vi "FL Get Rules as Text.vi"(8 "error in (no error)":errorcluster, 11 "fuzzy system in":T1 {"user MF interpolating polynomials"."coa_x(y) coeff" format="%.4g"; "user MF interpolating polynomials"."Area(y) coeff" format="%.4g"; "user MF interpolating polynomials"."X(y) coeff" format="%.4g"; "user MF interpolating polynomials"."Y(x) coeff" format="%.4g"; "user MF interpolating polynomials"."Y" format="%.4g"; "user MF interpolating polynomials"."X" format="%.4g"; "defuzzification method" items=["Center of Area", "Modified Center of Area", "Center of Sums", "Center of Maximum", "Mean of Maximum"]; "rules"."consequents"."Var Index" min=0; "rules"."consequents"."Cond" items=["=", "!="]; "rules"."consequents"."MF Index" min=0; "rules"."antecedents"."Var Index" min=0; "rules"."antecedents"."Cond" items=["=", "!="]; "rules"."antecedents"."MF Index" min=0; "rules"."consequent implication" items=["Minimum", "Product"]; "rules"."antecedent connective" items=["AND (Minimum)", "AND (Product)", "OR (Maximum)", "OR (Probabilistic)"]; "output variables"."MFs"."shape" items=["Triangle", "Trapezoid", "Singleton", "Sigmoid", "Gaussian", "User-Defined"]; "input variables"."MFs"."shape" items=["Triangle", "Trapezoid", "Singleton", "Sigmoid", "Gaussian", "User-Defined"]}) -> (0 "error out":errorcluster, 2 "rules as text":string[](array[string]), 3 "fuzzy system out":T1 {"user MF interpolating polynomials"."coa_x(y) coeff" format="%.4g"; "user MF interpolating polynomials"."Area(y) coeff" format="%.4g"; "user MF interpolating polynomials"."X(y) coeff" format="%.4g"; "user MF interpolating polynomials"."Y(x) coeff" format="%.4g"; "user MF interpolating polynomials"."Y" format="%.4g"; "user MF interpolating polynomials"."X" format="%.4g"; "defuzzification method" items=["Center of Area", "Modified Center of Area", "Center of Sums", "Center of Maximum", "Mean of Maximum"]; "rules"."consequents"."Var Index" min=0; "rules"."consequents"."Cond" items=["=", "!="]; "rules"."consequents"."MF Index" min=0; "rules"."antecedents"."Var Index" min=0; "rules"."antecedents"."Cond" items=["=", "!="]; "rules"."antecedents"."MF Index" min=0; "rules"."consequent implication" items=["Minimum", "Product"]; "rules"."antecedent connective" items=["AND (Minimum)", "AND (Product)", "OR (Maximum)", "OR (Probabilistic)"]; "output variables"."MFs"."shape" items=["Triangle", "Trapezoid", "Singleton", "Sigmoid", "Gaussian", "User-Defined"]; "input variables"."MFs"."shape" items=["Triangle", "Trapezoid", "Singleton", "Sigmoid", "Gaussian", "User-Defined"]})   [LabVIEW 2017, in "NI_Fuzzy_Logic_API.lvlib"]
doc: "Returns the rules of a fuzzy system in words."
uses:
  <vilib>/addons/Fuzzy Logic/NI_Fuzzy_Logic_API.lvlib
  <vilib>/addons/Fuzzy Logic/TypeDefs/FL System.ctl
  <vilib>/addons/Fuzzy Logic/TypeDefs/FL Variable.ctl
  <vilib>/addons/Fuzzy Logic/TypeDefs/FL Membership Function.ctl
  <vilib>/addons/Fuzzy Logic/TypeDefs/FL Membership Function Shape.ctl
  <vilib>/addons/Fuzzy Logic/TypeDefs/FL Rule.ctl
  <vilib>/addons/Fuzzy Logic/TypeDefs/FL Antecedent.ctl
  <vilib>/addons/Fuzzy Logic/TypeDefs/FL Modifier.ctl
  <vilib>/addons/Fuzzy Logic/TypeDefs/FL Antecedent Connective.ctl
  <vilib>/addons/Fuzzy Logic/TypeDefs/FL Consequent.ctl
  <vilib>/addons/Fuzzy Logic/TypeDefs/FL Consequent Implication.ctl
  <vilib>/addons/Fuzzy Logic/TypeDefs/FL Defuzzification.ctl
  <vilib>/addons/Fuzzy Logic/TypeDefs/FL Interpolating polynomials.ctl
panel:
  # "IF"
  # "THEN"
  # "IF"
  # "THEN"
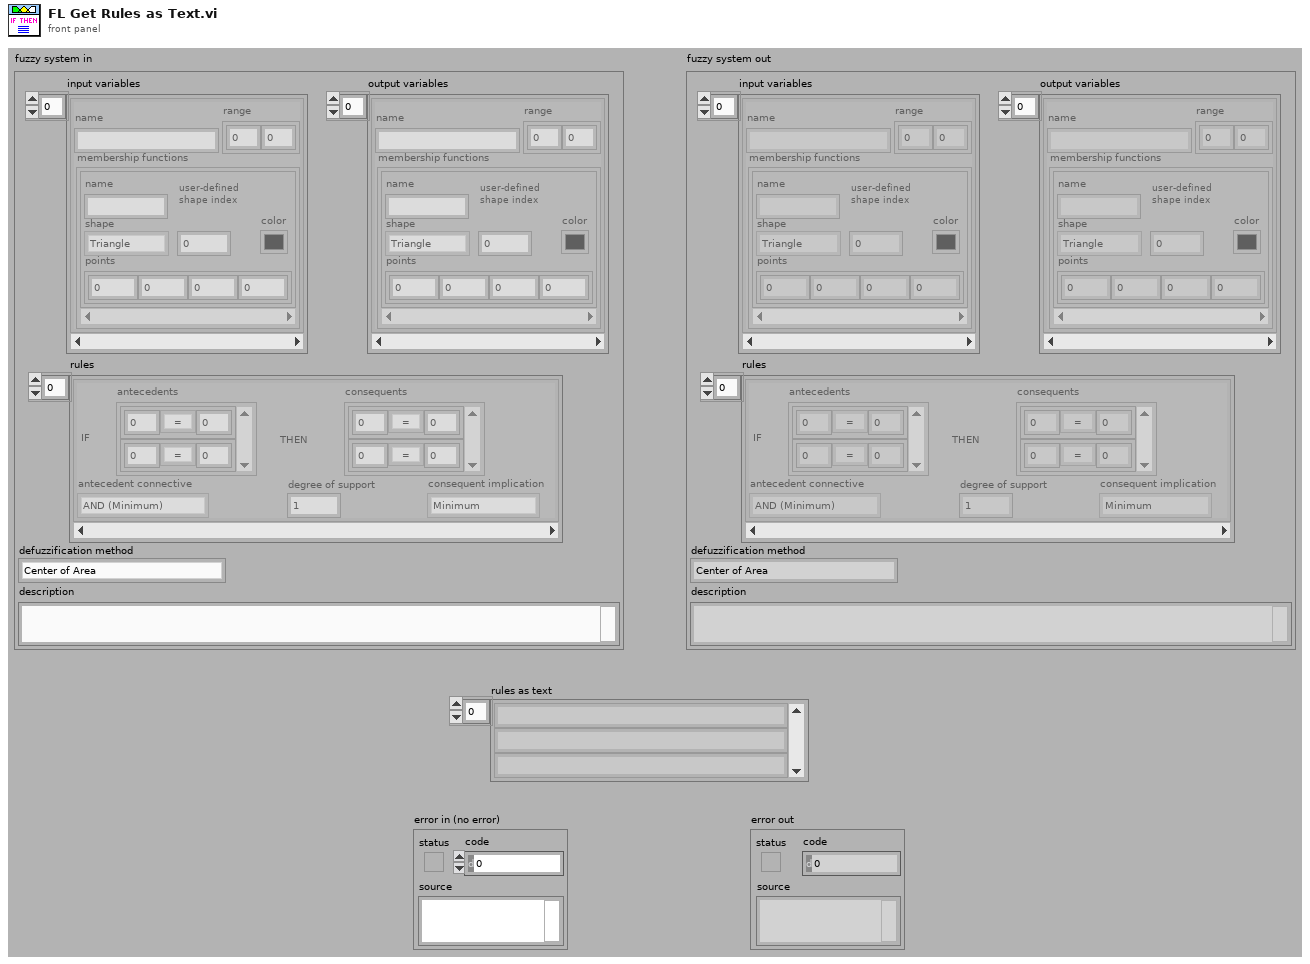
[diagram p1: front panel]
types:
  T1 = typedef "NI_Fuzzy_Logic_API.lvlib/FL System.ctl" = cluster{"input variables":T2[], "output variables":T2[], "rules":T5[], "defuzzification method":T11, "description":string, "user MF interpolating polynomials":T12[]}
  T2 = typedef "NI_Fuzzy_Logic_API.lvlib/FL Variable.ctl" = cluster{"name":string, "range":dbl[], "MFs":T3[]}
  T3 = typedef "NI_Fuzzy_Logic_API.lvlib/FL Membership Function.ctl" = cluster{"name":string, "shape":T4, "points":dbl[], "color":u32, "user-defined shape index":i32}
  T4 = typedef "NI_Fuzzy_Logic_API.lvlib/FL Membership Function Shape.ctl" = u16
  T5 = typedef "NI_Fuzzy_Logic_API.lvlib/FL Rule.ctl" = cluster{"antecedents":T6[], "antecedent connective":T8, "consequents":T9[], "consequent implication":T10, "degree of support":dbl}
  T6 = typedef "NI_Fuzzy_Logic_API.lvlib/FL Antecedent.ctl" = cluster{"Var Index":i32, "MF Index":i32, "Cond":T7}
  T7 = typedef "NI_Fuzzy_Logic_API.lvlib/FL Modifier.ctl" = u16
  T8 = typedef "NI_Fuzzy_Logic_API.lvlib/FL Antecedent Connective.ctl" = u16
  T9 = typedef "NI_Fuzzy_Logic_API.lvlib/FL Consequent.ctl" = cluster{"Var Index":i32, "MF Index":i32, "Cond":T7}
  T10 = typedef "NI_Fuzzy_Logic_API.lvlib/FL Consequent Implication.ctl" = u16
  T11 = typedef "NI_Fuzzy_Logic_API.lvlib/FL Defuzzification.ctl" = u16
  T12 = typedef "NI_Fuzzy_Logic_API.lvlib/FL Interpolating polynomials.ctl" = cluster{"X":dbl[], "Y":dbl[], "Y(x) coeff":dbl[][], "X(y) coeff":dbl[][], "Area(y) coeff":dbl[][], "coa_x(y) coeff":dbl[][]}
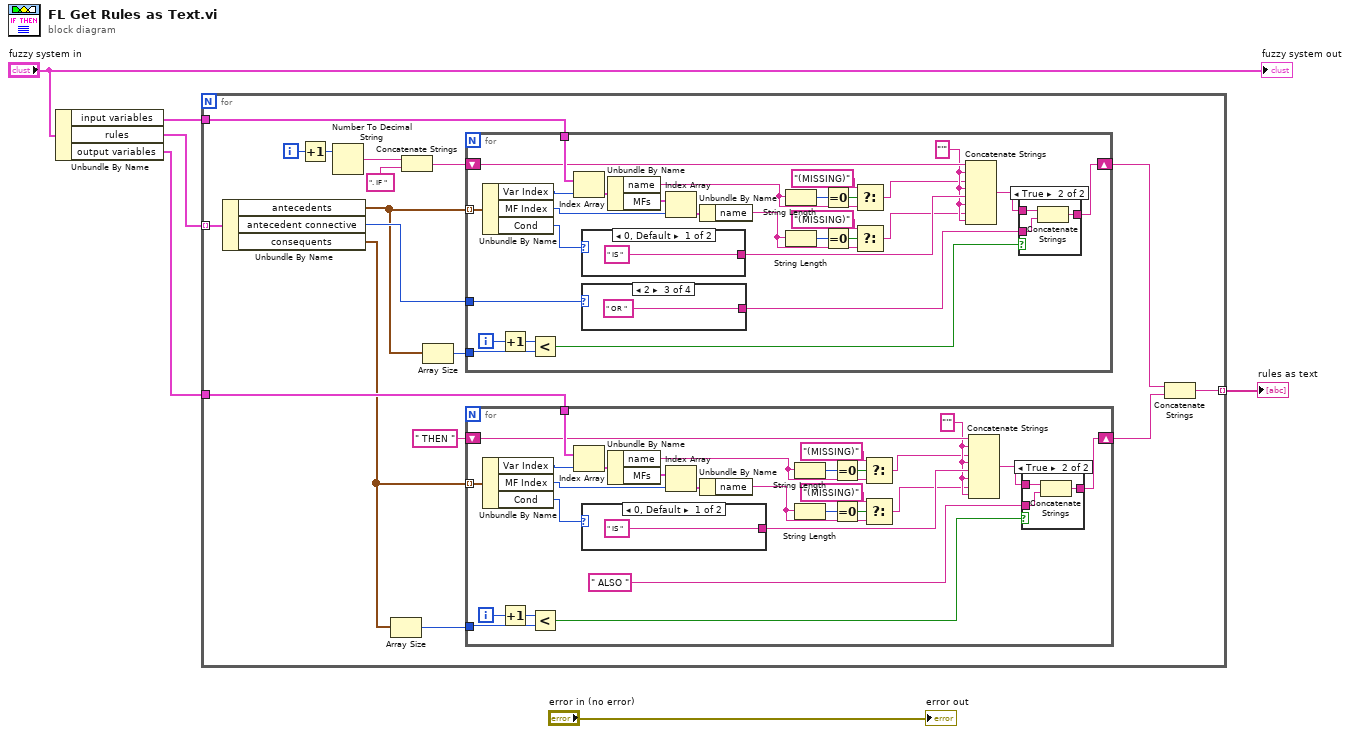
[diagram p0: block diagram]
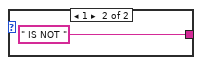
[diagram p3: hidden frame]
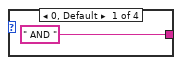
[diagram p5: hidden frame]
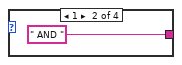
[diagram p6: hidden frame]
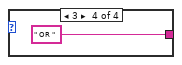
[diagram p7: hidden frame]
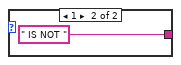
[diagram p8: hidden frame]
diagram:
  n1 = Unbundle By Name("fuzzy system in") -> ("input variables"=w3:T2[], "rules"=w2:T5[], "output variables"=w1:T2[])
  n2 = for {
    tunnel: w2 -> [w23] mode=indexing
    tunnel: w3 -> [w22]
    tunnel: w1 -> [w16]
    tunnel: [w12] -> w5 mode=indexing
    i -> [w8]
    n3 = Unbundle By Name(w23) -> ("antecedents"=w20:T6[], "antecedent connective"=w21:T8, "consequents"=w15:T9[])
    n4 = Increment(x=w8) -> (x+1=w7:i32)
    n5 = Number To Decimal String(number=w7) -> (decimal integer string=w11:string)  [unwired: 1 out]
    n6 = Array Size(array=w15) -> (size(s)=w17:i32)
    n7 = Concatenate Strings(w11, ". IF ") -> (w10:string)
    n8 = Array Size(array=w20) -> (size(s)=w19:i32)
    n9 = for {
      tunnel: w20 -> [w86] mode=indexing
      tunnel: w22 -> [w84]
      tunnel: w21 -> [w77]
      tunnel: w19 -> [w73]
      shift-right: [w70] -> w14
      shift-left: w10 -> [w69]
      i -> [w75]
      w68 = "'"
      n10 = Unbundle By Name(w86) -> ("Var Index"=w85:i32, "MF Index"=w81:i32, "Cond"=w79:T7)
      n11 = Increment(x=w75) -> (x+1=w74:i32)
      n12 = Less?(x=w74, y=w73) -> (x < y?=w71:bool)
      n13 = Index Array(array=w84, index=w85) -> (element=w83:T2)
      n14 = case shown="0, Default" w79 {
        tunnel: [" IS " ("string") " IS NOT " ("string")] -> w78
        frame 0, Default {
        }
        frame 1 {
        }
      }
      n15 = case shown="2" w77 {
        tunnel: [" AND " ("string") " AND " ("string") " OR " ("string") " OR " ("string")] -> w72
        frame 0, Default {
        }
        frame 1 {
        }
        frame 2 {
        }
        frame 3 {
        }
      }
      n16 = Unbundle By Name(w83) -> ("name"=w64:string, "MFs"=w82:T3[])
      n17 = Index Array(array=w82, index=w81) -> (element=w80:T3)
      n18 = Unbundle By Name(w80) -> ("name"=w59:string)
      n19 = String Length(string=w64) -> (length=w65:i32)
      n20 = String Length(string=w59) -> (length=w62:i32)
      n21 = Equal To 0?(x=w65) -> (x = 0?=w66:bool)
      n22 = Equal To 0?(x=w62) -> (x = 0?=w61:bool)
      n23 = Select(t="(MISSING)", s=w66, f=w64) -> (s? t:f=w63:string)
      n24 = Select(t="(MISSING)", s=w61, f=w59) -> (s? t:f=w58:string)
      n25 = Concatenate Strings(w69, w68, w63, w68, w78, w68, w58, w68) -> (w76:string)
      n26 = case shown="True" w71 {
        tunnel: w76 -> [w87 w90]
        tunnel: w72 -> [_ w89]
        tunnel: [w87 w88] -> w70
        frame False {
        }
        frame True {
          n27 = Concatenate Strings(w90, w89) -> (w88:string)
        }
      }
    }
    n28 = for {
      tunnel: w15 -> [w51] mode=indexing
      tunnel: w16 -> [w49]
      tunnel: w17 -> [w39]
      shift-right: [w36] -> w13
      shift-left: " THEN " -> [w35]
      i -> [w41]
      w34 = "'"
      n29 = Unbundle By Name(w51) -> ("Var Index"=w50:i32, "MF Index"=w46:i32, "Cond"=w44:T7)
      n30 = Increment(x=w41) -> (x+1=w40:i32)
      n31 = Less?(x=w40, y=w39) -> (x < y?=w37:bool)
      n32 = Index Array(array=w49, index=w50) -> (element=w48:T2)
      n33 = case shown="0, Default" w44 {
        tunnel: [" IS " ("string") " IS NOT " ("string")] -> w43
        frame 0, Default {
        }
        frame 1 {
        }
      }
      n34 = Unbundle By Name(w48) -> ("name"=w27:string, "MFs"=w47:T3[])
      n35 = Index Array(array=w47, index=w46) -> (element=w45:T3)
      n36 = Unbundle By Name(w45) -> ("name"=w25:string)
      n37 = String Length(string=w27) -> (length=w30:i32)
      n38 = String Length(string=w25) -> (length=w31:i32)
      n39 = Equal To 0?(x=w30) -> (x = 0?=w29:bool)
      n40 = Equal To 0?(x=w31) -> (x = 0?=w32:bool)
      n41 = Select(t="(MISSING)", s=w29, f=w27) -> (s? t:f=w26:string)
      n42 = Select(t="(MISSING)", s=w32, f=w25) -> (s? t:f=w24:string)
      n43 = Concatenate Strings(w35, w34, w26, w34, w43, w34, w24, w34) -> (w42:string)
      n44 = case shown="True" w37 {
        tunnel: w42 -> [w52 w55]
        tunnel: " ALSO " ("string") -> [_ w54]
        tunnel: [w52 w53] -> w36
        frame False {
        }
        frame True {
          n45 = Concatenate Strings(w55, w54) -> (w53:string)
        }
      }
    }
    n46 = Concatenate Strings(w14, w13) -> (w12:string)
  }
  "rules as text" <- w5
  "fuzzy system out" <- "fuzzy system in"
  "error out" <- "error in (no error)"
